vi "HEWH Adjust GPM.vi"(6 "Gallon Target":T1 format="%.2f", 7 "Equipment VISA":T2, 9 "GPM Target":T1 format="%.2f", 11 "Core HEWH Data in":T3={"Scan Rate Adjust"=0.0, "Draw Count"=0, "Test Patten Setup"={"Dispense Times"=[], "Total Gallons Schedule"=[], "Flow Rate Schedule "=[], "Incoming Water Temperature"=[], "PreDraw Pattern"=[], "24 Hour PreDraw"=enum."Zero Pre-Draws", "Pre-Draw Until?"=[], "Purge Until Cutout"=FALSE, "Heating Flag"=FALSE}, "Condition Cluster Output"={"Condition #1"=FALSE, "Condition #2"=FALSE, "Special Last Draw (HU Test)"=FALSE, "RTD Out Temperature <="=0.0, "Condition #3"=FALSE, "Mean Tank Temperature <="=0.0, "Condition #4"=FALSE, "Decrease Outlet Temperature \nBy (RTD Out)"=0.0, "Condition #5"=FALSE, "Condition #6"=FALSE, "Time (Seconds)"=0.0, "Condition #7"=FALSE, "Condition #8"=FALSE, "Draw Until Condition"={"UE"=FALSE, "LE"=FALSE, "COMP"=FALSE, "FANS"=FALSE}}, "HEWH Specific DAQ"={"HEWH Data"={"Voltage (Volts)"=0.0, "Current (Amps)"=0.0, "Power (Watts)"=0.0, "WattHours (Wh)"=0.0, "TC Tree (AVG)"=0.0, "Flow Rate (GPM)"=0.0, "Gallons (Gal)"=0.0, "RTD Out (Deg F)"=0.0, "TC Down"=0.0, "TC Tree Array"=[], "UE Event Lead"=0, "LE Event Lead"=0}, "Intellif Valve % Open"=0.0, "Power State"={"UE"=FALSE, "LE"=FALSE, "COMP"=FALSE, "FANS"=FALSE}, "Power Analyzer"=enum."APLUS", "Intellifaucet Configuration"=enum."DRK375,STATION3,1/2\"HOSE"}, "Test Output Data"={"PreDraw Data Table"=[], "Data Table"=[], "MW100 TC Headers"=[]}, "Calc and Calibration"={"RTD Max Min Array"=[], "Draw Statistics"=[], "Calibration Coefficients DBL"=[], "Min RTD Temp\nDuring Draw"=0.0, "Start Gallons"=0.0, "Starting Temp Decline Temp"=0.0, "Max RTD Temp\nDuring Draw"=0.0, "Draw Start Time"=0.0, "Delay Start Time"=0.0, "Current Purge Start Time"=0.0}, "Current Draw Time"=0.0} {"Test Patten Setup"."Incoming Water Temperature" format="%.2f"; "Test Patten Setup"."Flow Rate Schedule" format="%.2f"; "Test Patten Setup"."Total Gallons Schedule" format="%.2f"; "Test Patten Setup"."Dispense Times" format="%<%H:%M:%S>t"}) -> (0 "Custom Draw\nDispensed Gallons (Gal)":dbl, 2 "Core HEWH Data out":T3={"Scan Rate Adjust"=0.0, "Draw Count"=0, "Test Patten Setup"={"Dispense Times"=[], "Total Gallons Schedule"=[], "Flow Rate Schedule "=[], "Incoming Water Temperature"=[], "PreDraw Pattern"=[], "24 Hour PreDraw"=enum."Zero Pre-Draws", "Pre-Draw Until?"=[], "Purge Until Cutout"=FALSE, "Heating Flag"=FALSE}, "Condition Cluster Output"={"Condition #1"=FALSE, "Condition #2"=FALSE, "Special Last Draw (HU Test)"=FALSE, "RTD Out Temperature <="=0.0, "Condition #3"=FALSE, "Mean Tank Temperature <="=0.0, "Condition #4"=FALSE, "Decrease Outlet Temperature \nBy (RTD Out)"=0.0, "Condition #5"=FALSE, "Condition #6"=FALSE, "Time (Seconds)"=0.0, "Condition #7"=FALSE, "Condition #8"=FALSE, "Draw Until Condition"={"UE"=FALSE, "LE"=FALSE, "COMP"=FALSE, "FANS"=FALSE}}, "HEWH Specific DAQ"={"HEWH Data"={"Voltage (Volts)"=0.0, "Current (Amps)"=0.0, "Power (Watts)"=0.0, "WattHours (Wh)"=0.0, "TC Tree (AVG)"=0.0, "Flow Rate (GPM)"=0.0, "Gallons (Gal)"=0.0, "RTD Out (Deg F)"=0.0, "TC Down"=0.0, "TC Tree Array"=[], "UE Event Lead"=0, "LE Event Lead"=0}, "Intellif Valve % Open"=0.0, "Power State"={"UE"=FALSE, "LE"=FALSE, "COMP"=FALSE, "FANS"=FALSE}, "Power Analyzer"=enum."APLUS", "Intellifaucet Configuration"=enum."DRK375,STATION3,1/2\"HOSE"}, "Test Output Data"={"PreDraw Data Table"=[], "Data Table"=[], "MW100 TC Headers"=[]}, "Calc and Calibration"={"RTD Max Min Array"=[], "Draw Statistics"=[], "Calibration Coefficients DBL"=[], "Min RTD Temp\nDuring Draw"=0.0, "Start Gallons"=0.0, "Starting Temp Decline Temp"=0.0, "Max RTD Temp\nDuring Draw"=0.0, "Draw Start Time"=0.0, "Delay Start Time"=0.0, "Current Purge Start Time"=0.0}, "Current Draw Time"=0.0} {"Test Patten Setup"."Incoming Water Temperature" format="%.2f"; "Test Patten Setup"."Flow Rate Schedule" format="%.2f"; "Test Patten Setup"."Total Gallons Schedule" format="%.2f"; "Test Patten Setup"."Dispense Times" format="%<%H:%M:%S>t"})   [LabVIEW 2014]
uses:
  Type Definitions/HEWH Output Information.ctl
  Type Definitions/HEWH Draw Pattern Setup.ctl
  Type Definitions/HEWH PreDraw.ctl
  Type Definitions/HEWH Termination Condition Cluster.ctl
  Type Definitions/HEWH Power Elements.ctl
  Type Definitions/HEWH Power Data.ctl
  Utility/Type Definitions/UTILITY Power Analyzer.ctl
  Type Definitions/HEWH Intellifaucet Tested Flowrate Scenarios.ctl
  Type Definitions/HEWH Equipment References.ctl
  Utility/Custom Pallet Controls/Custom Pallet DBL.ctl
panel:
  # "Select Only One Condition"
  # "Just Draw Water!"
  # "Condition #1"
  # "Condition #2"
  # "Start Dispense Pattern"
  # "Draw Until Any Heat Source"
  # "Condition #3"
  # "Draw Until Specific Heat Source"
  # "Not Working"
  # "Condition #4"
  # "Condition #5"
  # "Condition #6"
  # "Draw Pattern Setup"
  # "Pre-Draw Items"
  # "Select Only One Condition"
  # "Just Draw Water!"
  # "Condition #1"
  # "Condition #2"
  # "Start Dispense Pattern"
  # "Draw Until Any Heat Source"
  # "Condition #3"
  # "Draw Until Specific Heat Source"
  # "Not Working"
  # "Condition #4"
  # "Condition #5"
  # "Condition #6"
  # "Draw Pattern Setup"
  # "Pre-Draw Items"
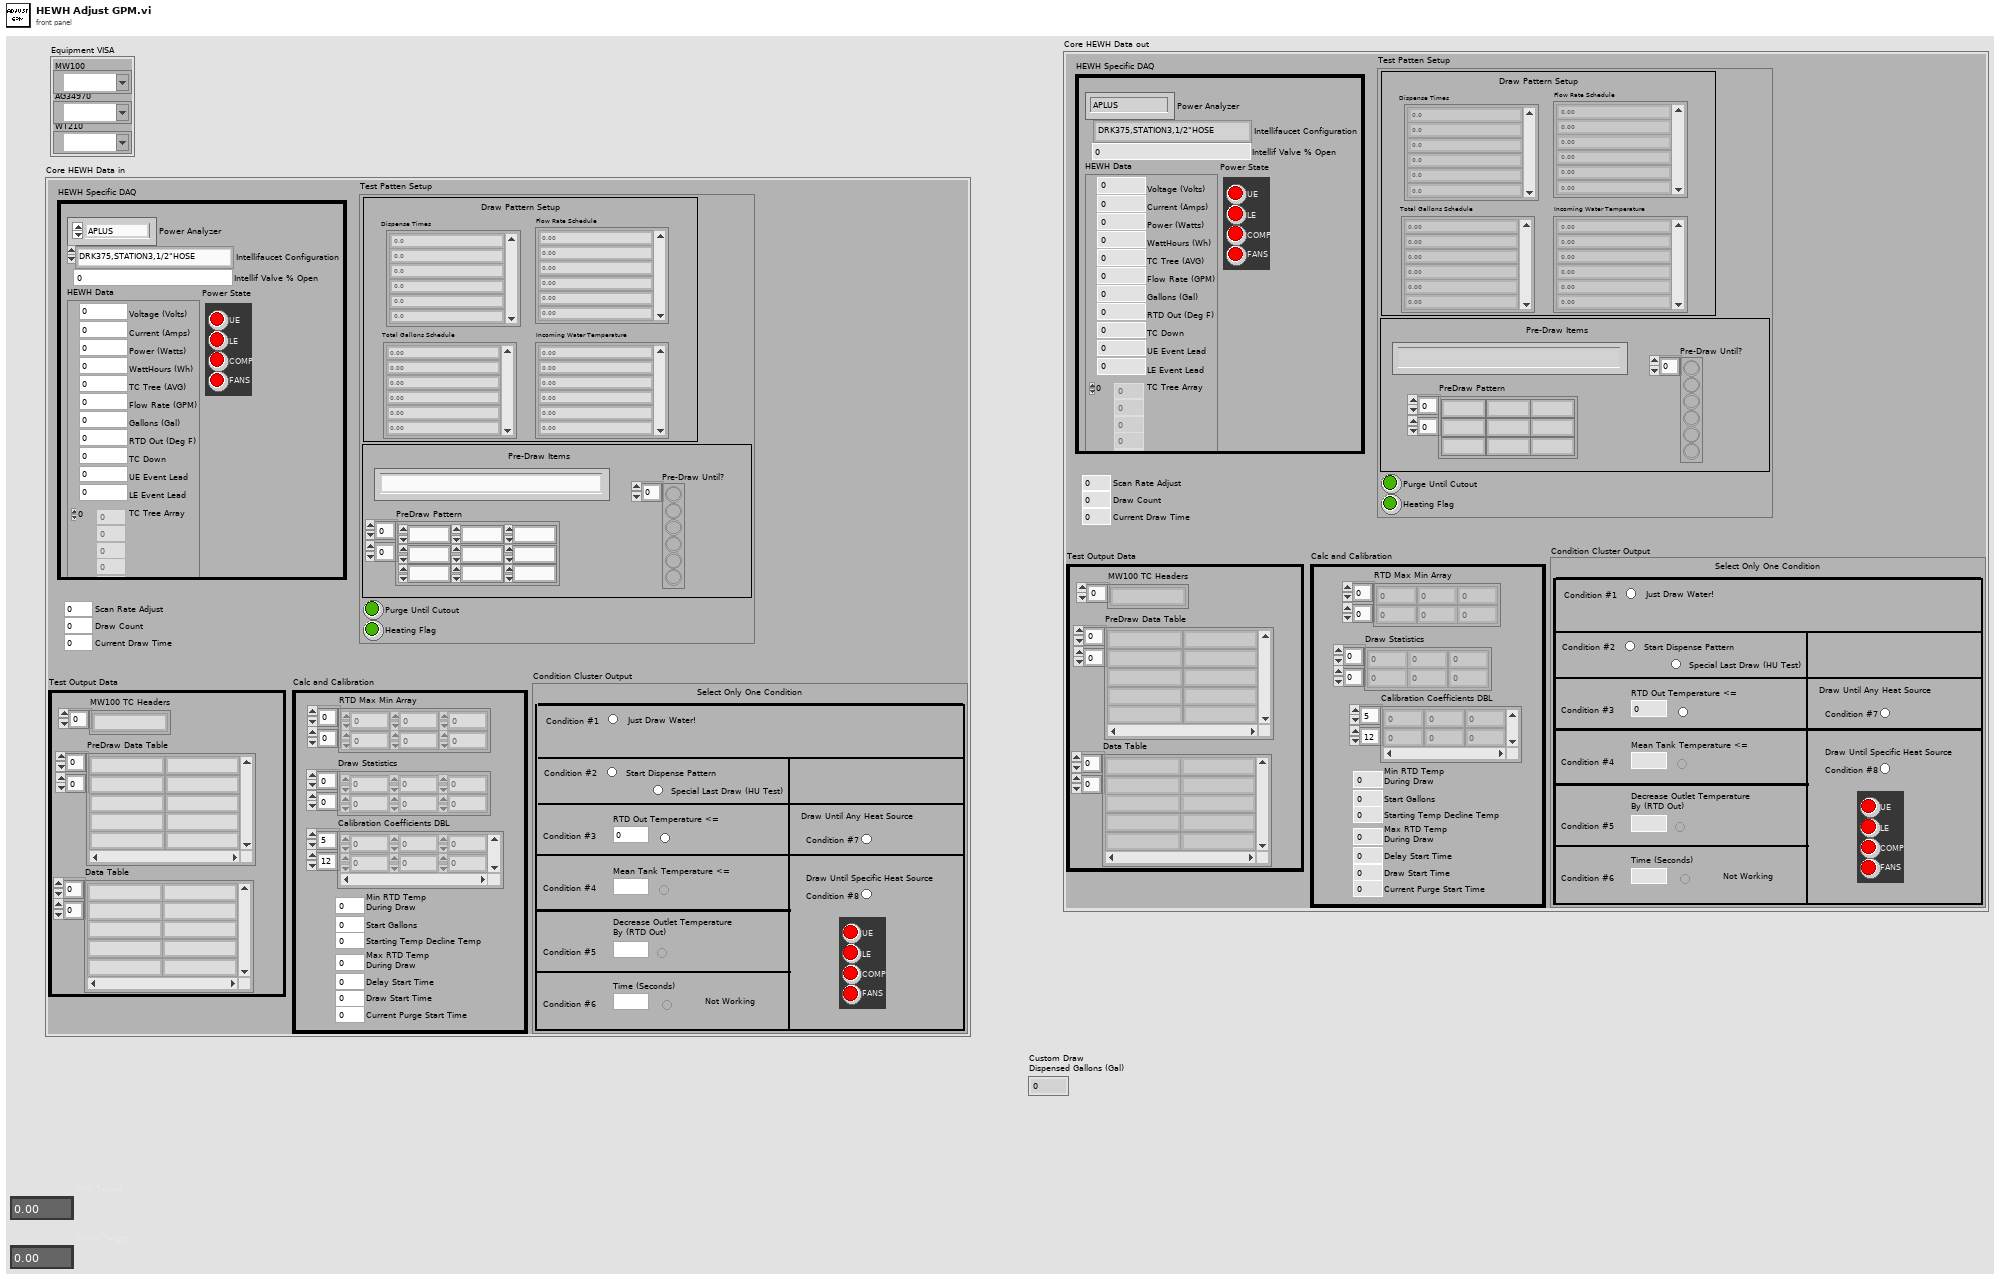
[diagram p1: front panel]
types:
  T1 = typedef "Custom Pallet DBL.ctl" = dbl
  T2 = typedef "HEWH Equipment References.ctl" = cluster{"MW100":refnum<visa-resource-name>, "AG34970":refnum<visa-resource-name>, "WT210":refnum<visa-resource-name>}
  T3 = typedef "HEWH Output Information.ctl" = cluster{"Scan Rate Adjust":dbl, "Draw Count":i32, "Test Patten Setup":T4, "Condition Cluster Output":T6, "HEWH Specific DAQ":cluster{"HEWH Data":T8, "Intellif Valve % Open":dbl, "Power State":T7, "Power Analyzer":T9, "Intellifaucet Configuration":T10}, "Test Output Data":cluster{"PreDraw Data Table":string[][], "Data Table":string[][], "MW100 TC Headers":string[]}, "Calc and Calibration":cluster{"RTD Max Min Array":dbl[][], "Draw Statistics":dbl[][], "Calibration Coefficients DBL":dbl[][], "Min RTD Temp\nDuring Draw":dbl, "Start Gallons":dbl, "Starting Temp Decline Temp":dbl, "Max RTD Temp\nDuring Draw":dbl, "Draw Start Time":dbl, "Delay Start Time":dbl, "Current Purge Start Time":dbl}, "Current Draw Time":dbl}
  T4 = typedef "HEWH Draw Pattern Setup.ctl" = cluster{"Dispense Times":dbl[], "Total Gallons Schedule":dbl[], "Flow Rate Schedule ":dbl[], "Incoming Water Temperature":dbl[], "PreDraw Pattern":dbl[][], "24 Hour PreDraw":T5, "Pre-Draw Until?":bool[], "Purge Until Cutout":bool, "Heating Flag":bool}
  T5 = typedef "HEWH PreDraw.ctl" = enum16{"Zero Pre-Draws", "One Pre- Draws", "Two Pre-Draws", "Three Pre-Draws", ""}
  T6 = typedef "HEWH Termination Condition Cluster.ctl" = cluster{"Condition #1":bool, "Condition #2":bool, "Special Last Draw (HU Test)":bool, "RTD Out Temperature <=":dbl, "Condition #3":bool, "Mean Tank Temperature <=":dbl, "Condition #4":bool, "Decrease Outlet Temperature \nBy (RTD Out)":dbl, "Condition #5":bool, "Condition #6":bool, "Time (Seconds)":dbl, "Condition #7":bool, "Condition #8":bool, "Draw Until Condition":T7}
  T7 = typedef "HEWH Power Elements.ctl" = cluster{"UE":bool, "LE":bool, "COMP":bool, "FANS":bool}
  T8 = typedef "HEWH Power Data.ctl" = cluster{"Voltage (Volts)":dbl, "Current (Amps)":dbl, "Power (Watts)":dbl, "WattHours (Wh)":dbl, "TC Tree (AVG)":dbl, "Flow Rate (GPM)":dbl, "Gallons (Gal)":dbl, "RTD Out (Deg F)":dbl, "TC Down":dbl, "TC Tree Array":dbl[], "UE Event Lead":i32, "LE Event Lead":i32}
  T9 = typedef "UTILITY Power Analyzer.ctl" = enum16{"", "APLUS", "WT210", "WT500", "WT300", "OSI", "Debug"}
  T10 = typedef "HEWH Intellifaucet Tested Flowrate Scenarios.ctl" = enum16{"DRK500,Station1", "DRK375,Lab", "SRK500,Station1,5GPM FR", "DRK375,STATION3,1/2\"HOSE", "DRK500,Station1,downspout", "DRK375,Station3,thruEcocute", "DRK375,Station3,purge", "Build2,2B,Purge", "Global, Purge", "Global, Tank", "DRK250"}
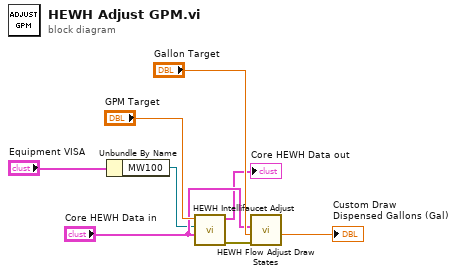
[diagram p0: block diagram]
diagram:
  n1 = Unbundle By Name("Equipment VISA") -> ("MW100"=w1:refnum<visa-resource-name>)
  n2 = call "HEWH Intellifaucet Adjust.vi"("Core HEWH Data in"="Core HEWH Data in", "MW100"=w1, "GPM Target"="GPM Target") -> ("error out"=w3:errorcluster, "Core HEWH Data out"=→"Core HEWH Data out":T3)  [unwired: 7 in]
  n3 = call "HEWH Flow Adjust Draw States.vi"("Error In"=w3, "Gallon Target"="Gallon Target", "Core HEWH Data in"="Core HEWH Data in") -> ("Custom Draw\nDispensed Gallons (Gal)"=→"Custom Draw\nDispensed Gallons (Gal)":dbl)  [unwired: 6 in, 2 out]
